vi "Variable list Driller analog.vi"() -> (6 "Variant":variant, 10 "Array":T1[](array[typedef]) {"Default Scaling"."Offset" format="%.5f"; "Default Scaling"."Gain" format="%.5f"})   [LabVIEW 2011]
uses:
  Measurments Handling/Fixed Analog Channel Definition.ctl
  Measurments Handling/Units/Quantity enum.ctl
  Measurments Handling/Update frequensies.ctl
  Measurments Handling/Channel catagory Enum.ctl
  Measurments Handling/Scaling.ctl
  Variable List Driller Analog.ctl
  <vilib>/Utility/VariantDataType/GetNumericInfo.vi
panel:
  in  "String":string
  out "Text Elements":string[](array[string])
  # "tool motor rpm"
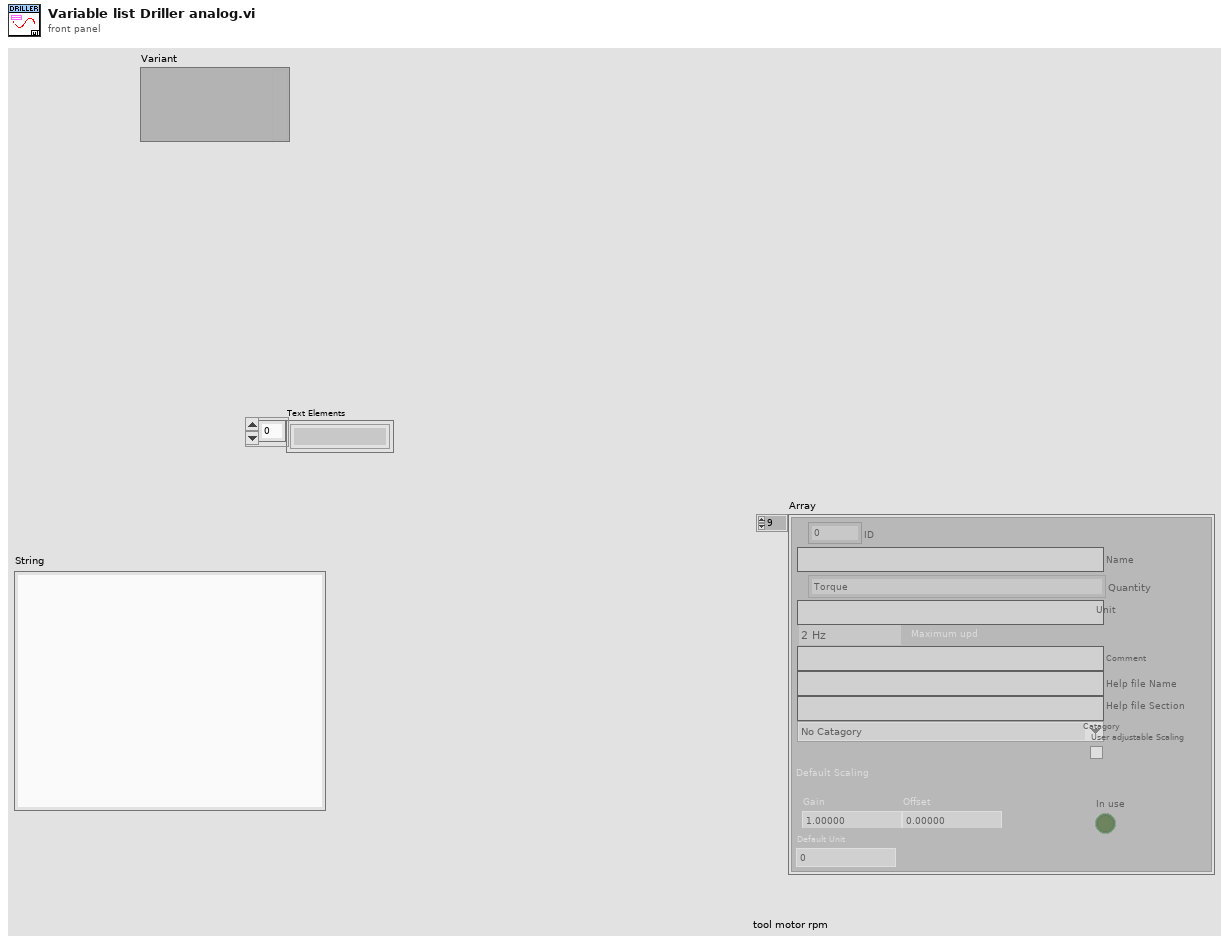
[diagram p1: front panel]
types:
  T1 = typedef "Fixed Analog Channel Definition.ctl" = cluster{"ID":u16, "Name":string, "Quantity":T2, "Unit":string, "Maximum upd":T3, "Comment":string, "Help file Name":string, "Help file Section ":string, "Catagory":T4, "User adjustable Scaling":bool, "Default Scaling":T5, "In use":bool, "Default Unit":i32}
  T2 = typedef "Quantity enum.ctl" = enum16{"Acceleration", "Angle", "Current", "Force", "Distance", "Pressure", "Resistance", "Rotational Speed", "Speed", "Temperature", "Tension", "Torque", "Voltage", "Weight"}
  T3 = typedef "Update frequensies.ctl" = enum16{"2 Hz", "1 Hz", "0.1 Hz"}
  T4 = typedef "Channel catagory Enum.ctl" = enum16{"No Catagory", "Power", "Temperature", "Pressure"}
  T5 = typedef "Scaling.ctl" = cluster{"Gain":dbl, "Offset":dbl}
  T6 = typedef "Variable List Driller Analog.ctl" = enum16{"Tool max Temperature", "Tool (Solenoid) Temperature", "Tool supply Voltage", "Tool (Controller) Current", "Tool Acceleration X", "Tool Acceleration Y", "Tool Acceleration Z", "Tool (Controller) Temperature", "Tool Acceleration Sum", "Tool Inclination", "Tool Rotation", "Tool GP Sensor 1", "Tool GP Sensor 2", "Tool (Pressure 1) Temperature", "Tool Pressure 1", "Tool (Pressure 2) Temperature", "Tool Pressure 2", "Tool Motor Voltage", "Tool Motor Current", "Tool Motor Torque", "Tool Temperature sensor", "Tool weight on bit", "Tool Motor RPM", "PSU Temp", "PSU HV Voltage in", "PSU Main Voltage out", "PSU Main Current out"}
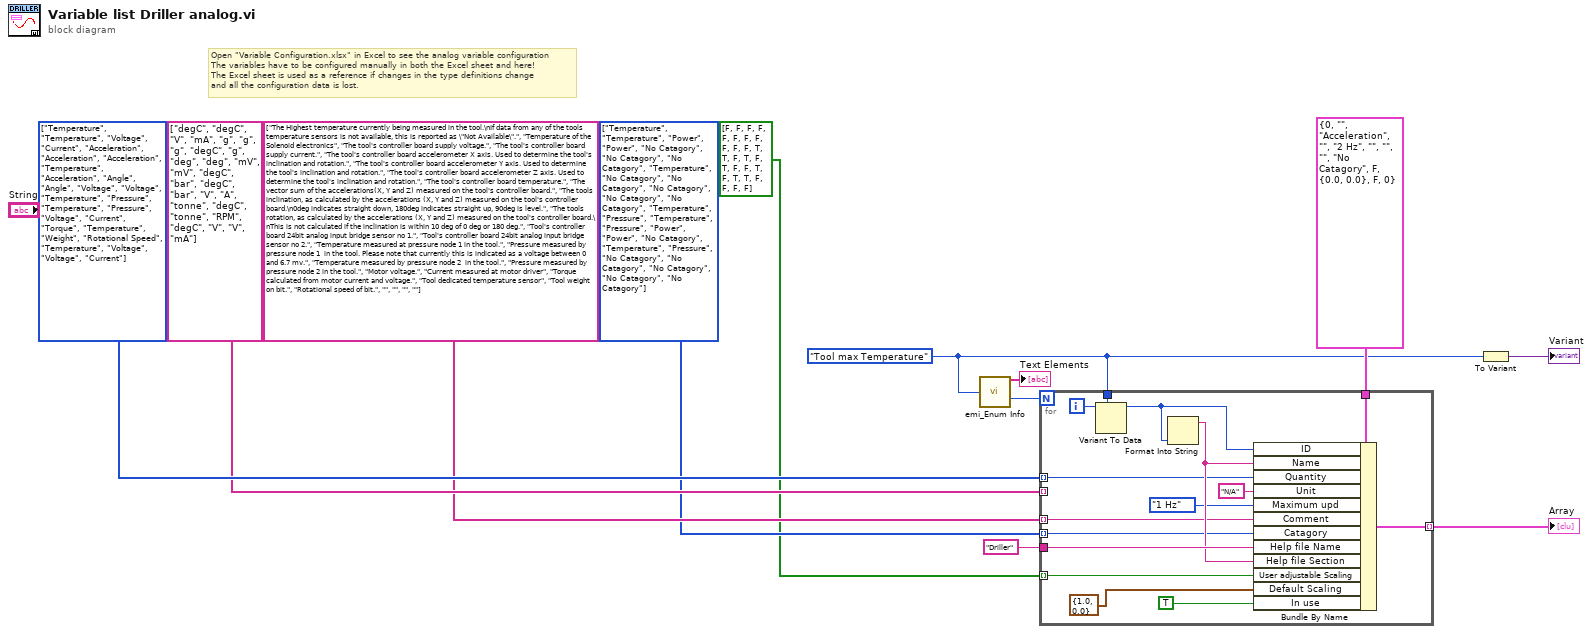
[diagram p0: block diagram]
diagram:
  w4 = T4[] [enum."Temperature", enum."Temperature", enum."Power", enum."Power", enum."No Catagory", enum."No Catagory", enum."No Catagory", enum."Temperature", enum."No Catagory", enum."No Catagory", enum."No Catagory", enum."No Catagory", enum."No Catagory", enum."Temperature", enum."Pressure", enum."Temperature", enum."Pressure", enum."Power", enum."Power", enum."No Catagory", enum."Temperature", enum."Pressure", enum."No Catagory", enum."No Catagory", enum."No Catagory", enum."No Catagory", enum."No Catagory"] items=["No Catagory", "Power", "Temperature", "Pressure"]
  w7 = T2[] [enum."Temperature", enum."Temperature", enum."Voltage", enum."Current", enum."Acceleration", enum."Acceleration", enum."Acceleration", enum."Temperature", enum."Acceleration", enum."Angle", enum."Angle", enum."Voltage", enum."Voltage", enum."Temperature", enum."Pressure", enum."Temperature", enum."Pressure", enum."Voltage", enum."Current", enum."Torque", enum."Temperature", enum."Weight", enum."Rotational Speed", enum."Temperature", enum."Voltage", enum."Voltage", enum."Current"] items=["Acceleration", "Angle", "Current", "Force", "Distance", "Pressure", "Resistance", "Rotational Speed", "Speed", "Temperature", "Tension", "Torque", "Voltage", "Weight"]
  w8 = Variable_List_Driller_Analog."Tool max Temperature" ("Action")
  # "Open \"Variable Configuration.xlsx\" in Excel to see the analog variable configuration\nThe variables have to be configured manually in both the Excel sheet and here!\nThe Excel sheet is used as a reference if changes in the type definitions change\nand all the configuration data is lost."
  n1 = call "emi_Enum Info.vi"("Enum"=w8) -> ("Text Elements"=→"Text Elements":string[], "Numb Elements"=w9:i32)  [unwired: 11 in, 2 out]
  n2 = for {
    N: w9 -> [_]
    tunnel: "Driller" ("Help file Name") -> [w23]
    tunnel: [w27] -> w2 mode=indexing
    tunnel: T1 {"ID"=0, "Name"="", "Quantity"=enum."Acceleration", "Unit"="", "Maximum upd"=enum."2 Hz", "Comment"="", "Help file Name"="", "Help file Section "="", "Catagory"=enum."No Catagory", "User adjustable Scaling"=FALSE, "Default Scaling"={"Gain"=0.0, "Offset"=0.0}, "In use"=FALSE, "Default Unit"=0} ("Variable Defenition") -> [w26]
    tunnel: w8 -> [w21]
    tunnel: w7 -> [w18] mode=indexing
    tunnel: string[] ["degC", "degC", "V", "mA", "g", "g", "g", "degC", "g", "deg", "deg", "mV", "mV", "degC", "bar", "degC", "bar", "V", "A", "tonne", "degC", "tonne", "RPM", "degC", "V", "V", "mA"] -> [_] mode=indexing
    tunnel: string[] ["The Highest temperature currently being measured in the tool.\nIf data from any of the tools temperature sensors is not available, this is reported as \"Not Available\".", "Temperature of the Solenoid electronics", "The tool's controller board supply voltage.", "The tool's controller board supply current.", "The tool's controller board accelerometer X axis. Used to determine the tool's inclination and rotation.", "The tool's controller board accelerometer Y axis. Used to determine the tool's inclination and rotation.", "The tool's controller board accelerometer Z axis. Used to determine the tool's inclination and rotation.", "The tool's controller board temperature.", "The vector sum of the accelerations(X, Y and Z) measured on the tool's controller board.", "The tools inclination, as calculated by the accelerations (X, Y and Z) measured on the tool's controller board.\n0deg indicates straight down, 180deg indicates straight up, 90deg is level.", "The tools rotation, as calculated by the accelerations (X, Y and Z) measured on the tool's controller board.\nThis is not calculated if the inclination is within 10 deg of 0 deg or 180 deg.", "Tool's controller board 24bit analog input bridge sensor no 1.", "Tool's controller board 24bit analog input bridge sensor no 2.", "Temperature measured at pressure node 1 in the tool.", "Pressure measured by pressure node 1  in the tool. Please note that currently this is indicated as a voltage between 0 and 6.7 mv.", "Temperature measured by pressure node 2  in the tool.", "Pressure measured by pressure node 2 in the tool.", "Motor voltage.", "Current measured at motor driver", "Torque calculated from motor current and voltage.", "Tool dedicated temperature sensor", "Tool weight on bit.", "Rotational speed of bit.", "", "", "", ""] -> [w16] mode=indexing
    tunnel: w4 -> [w15] mode=indexing
    tunnel: bool[] [FALSE, FALSE, FALSE, FALSE, FALSE, FALSE, FALSE, FALSE, FALSE, FALSE, FALSE, TRUE, TRUE, FALSE, TRUE, FALSE, TRUE, FALSE, FALSE, TRUE, FALSE, TRUE, TRUE, FALSE, FALSE, FALSE, FALSE] -> [w14] mode=indexing
    i -> [w22]
    n3 = Variant To Data(type=w21, Variant=w22) -> (data=w20:T6)  [unwired: 1 in, 1 out]
    n4 = Format Into String(w20) -> (resulting string=w19:string)  [unwired: 3 in, 1 out]
    n5 = Bundle By Name(cluster=w26, "ID"=w20, "Name"=w19, "Quantity"=w18, "Unit"="N/A", "Maximum upd"=Update_frequensies."1 Hz", "Comment"=w16, "Catagory"=w15, "Help file Name"=w23, "Help file Section"=w19, "User adjustable Scaling"=w14, "Default Scaling"=T5 {"Gain"=1.0, "Offset"=0.0}, "In use"=TRUE ("Variable Defenition.In use")) -> (w27:T1)
  }
  "Array" <- w2
  n6 = To Variant(anything=w8) -> (Variant=→"Variant":variant)
